vi "niRFUtil MASMT Decimate (single shot) (DBL).vi"(8 "error in (no error)":errorcluster, 9 "averaging":bool, 10 "decimating factor":i32=1, 11 "X":dbl[](array[numeric])) -> (0 "error out":errorcluster, 3 "Decimated X":dbl[](array[numeric]))   [LabVIEW 2015, in "niRFUtil.lvlib"]
doc: "Decimates the input sequence <B>X</B> by the <B>decimating factor</B>."
uses:
  niRFUtil.lvlib
  Utilities/niRFMASMT_FFT.dll
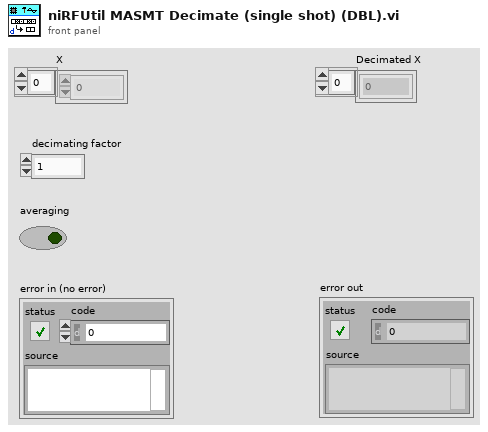
[diagram p1: front panel]
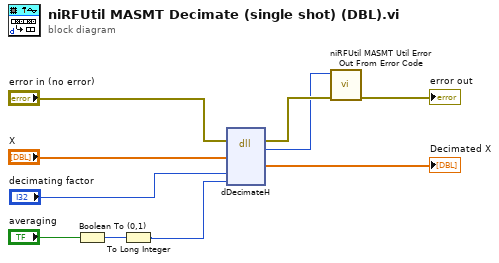
[diagram p0: block diagram]
diagram:
  n1 = Boolean To (0,1)(Boolean="averaging") -> (0, 1=w3:i16)
  n2 = To Long Integer(number=w3) -> (32bit integer=w2:i32)
  n3 = dll-call lib="C:/Perforce/semoore-sales/Customers/NATI-3813/Noise Floor/LV Filters/ParallelComplexFilterRFUtil/niRFUtil/MASMT/Utilities/niRFMASMT_FFT.*" fn="dDecimateH"(error in="error in (no error)", "xH"="X", "factor"="decimating factor", "average"=w2) -> (error out=w8:errorcluster, "return type"=w7:i32, "yH"=→"Decimated X":dbl[])  [unwired: 6 in, 1 out]
  n4 = call "niRFUtil MASMT Util Error Out From Error Code.vi"("error in (no error)"=w8, "error code"=w7) -> ("error out"=→"error out":errorcluster)  [unwired: 9 in]
